vi "Mag_Phase_Calculator (SubVI).vi"(7 "even-angle references":cluster{"r0":dbl, "dr":dbl, "Y":dbl[]}[](array[cluster]) {"r0" format="%.2p"; "dr" format="%.2p"; "Y" format="%.2f"}, 8 "error in (no error)":errorcluster, 9 "view":T2={"dB on? (F)"=FALSE, "unwrap phase? (T)"=TRUE, "unit in degree? (T)"=TRUE}, 10 "speed profile":T1 {"speed [RPM]" format="%.2f"; "time [s]" format="%.2f"}, 11 "Array in":waveform(dbl)[](array[waveform])) -> (0 "error out":errorcluster, 1 "Computed Mag/Phase":cluster{dbl, dbl, dbl, dbl}[](array[cluster]), 2 "RPS (Hz)":dbl, 3 "Data Available":bool)   [LabVIEW 2012]
uses:
  <vilib>/addons/Sound and Vibration/Order Analysis/Tach Process/SubVIs/speed profile.ctl
  <vilib>/addons/Sound and Vibration/Order Analysis/Referece Data Processing/OAT Compensate Even Angle Signal (Even Angle Ref, N Channels).vi
  <vilib>/addons/Sound and Vibration/Order Analysis/Resample Order Tracking/SoundVib_OrderTracking.lvlib
  <vilib>/addons/Sound and Vibration/Order Analysis/Referece Data Processing/SoundVib_RefDataProcess.lvlib
  <vilib>/addons/Sound and Vibration/Order Analysis/Tach Process/SoundVib_TachProcess.lvlib
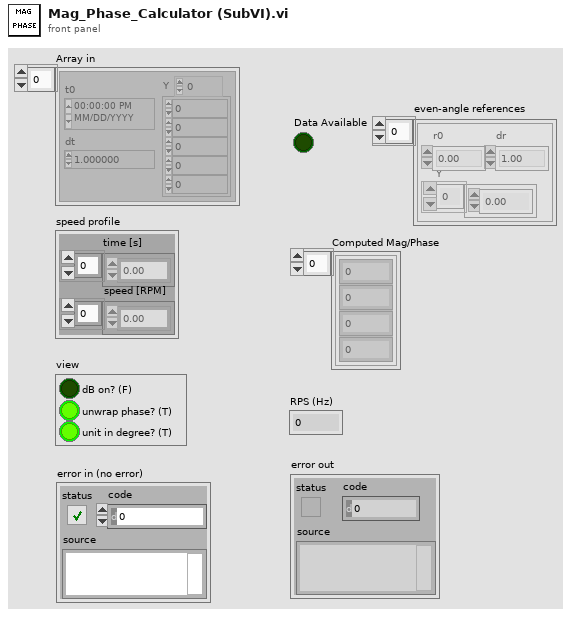
[diagram p1: front panel]
types:
  T1 = typedef "SoundVib_TachProcess.lvlib/speed profile.ctl" = cluster{"time [s]":dbl[], "speed [RPM]":dbl[]}
  T2 = cluster{"dB on? (F)":bool, "unwrap phase? (T)":bool, "unit in degree? (T)":bool}
  T3 = typedef "svc_Resampled Channel Info.ctl" = cluster{"channel name":string, "description":string, " channel info":T4}
  T4 = typedef "svc_Channel Info.ctl" = cluster{"sensor sensitivity [mV/EU]":dbl, "engineering units":T5, "dB reference [EU]":dbl, "custom label":string, "weighting filter":T6, "pregain [dB]":dbl}
  T5 = typedef "svc_Engineering Units Text Ring.ctl" = u16
  T6 = typedef "svc_Weighting Filter Text Ring.ctl" = u16
  T7 = typedef "OAT Position Info.ctl" = cluster{"positions [s]":dbl[], "samples/rev":dbl}
  T8 = cluster{"time/rev/rpm":dbl[], "magnitude":dbl[]}[][]
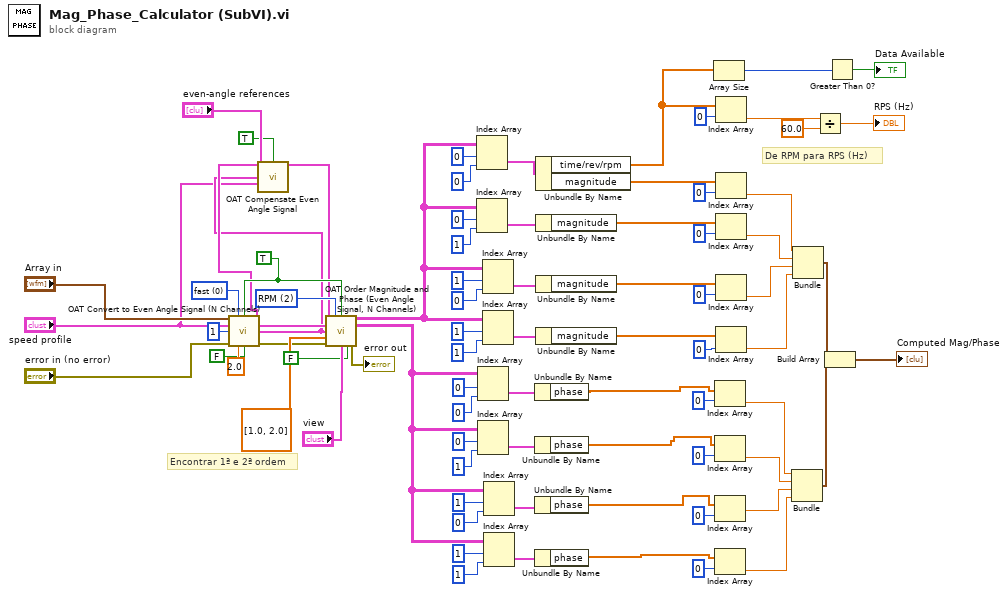
[diagram p0: block diagram]
diagram:
  w79 = TRUE
  w28 = u16 0 items=["fast", "accurate"] ("analysis method")
  w23 = u16 2 items=["Time", "Revolution", "RPM"] ("X axis selection")
  # "Encontrar 1ª e 2ª ordem"
  # "De RPM para RPS (Hz)"
  n1 = call <vilib>:"OAT Convert to Even Angle Signal (N Channels).vi"("scaled signals [EU]"="Array in", "analysis method"=w28, "reset? (F)"=w79, "speed profile"="speed profile", "pulse/revolution (1)"=1, "error in (no error)"="error in (no error)", "max order (auto)"=2.0, "zero delay? (F)"=FALSE) -> ("even-angle signals"=w13:cluster{"r0":dbl, "dr":dbl, "Y":dbl[]}[], "even-angle channel info"=w22:T3[], "even-angle position info"=w11:T7, "error out"=w27:errorcluster)  [unwired: 3 in, 1 out]
  n2 = call-poly <vilib>:"OAT Compensate Even Angle Signal.vi"("even-angle signals"=w13, "reset? (F)"=TRUE, "even-angle references"="even-angle references", "even-angle position info"=w11, "speed profile"="speed profile") -> ("compensated even-angle signals"=w12:cluster{"r0":dbl, "dr":dbl, "Y":dbl[]}[])  [unwired: 7 in, 3 out]
  n3 = call <vilib>:"OAT Order Magnitude and Phase (Even Angle Signal, N Channels).vi"("even-angle signals"=w12, "x-axis selection"=w23, "reset? (F)"=w79, "even-angle channel info"=w22, "even-angle position info"=w11, "orders to compute (1.0)"=dbl[] [1.0, 2.0], "error in (no error)"=w27, "view"="view", "zero delay? (F)"=FALSE) -> ("magnitudes [RMS]"=w3:T8, "phases [phase lag]"=w2:cluster{"time/rev/rpm":dbl[], "phase":dbl[]}[][], "error out"=→"error out":errorcluster)  [unwired: 1 in, 3 out]
  n4 = Index Array(array=w3, index (row)=0, index (col)=0 ("index (row)")) -> (element=w32:cluster{"time/rev/rpm":dbl[], "magnitude":dbl[]})
  n5 = Index Array(array=w3, index (row)=0, index (col)=1 ("index (row)")) -> (element=w35:cluster{"time/rev/rpm":dbl[], "magnitude":dbl[]})
  n6 = Index Array(array=w2, index (row)=0, index (col)=0 ("index (row)")) -> (element=w48:cluster{"time/rev/rpm":dbl[], "phase":dbl[]})
  n7 = Index Array(array=w2, index (row)=0, index (col)=1 ("index (row)")) -> (element=w8:cluster{"time/rev/rpm":dbl[], "phase":dbl[]})
  n8 = Index Array(array=w3, index (row)=1, index (col)=0 ("index (row)")) -> (element=w37:cluster{"time/rev/rpm":dbl[], "magnitude":dbl[]})
  n9 = Index Array(array=w3, index (row)=1, index (col)=1 ("index (row)")) -> (element=w40:cluster{"time/rev/rpm":dbl[], "magnitude":dbl[]})
  n10 = Index Array(array=w2, index (row)=1, index (col)=0 ("index (row)")) -> (element=w44:cluster{"time/rev/rpm":dbl[], "phase":dbl[]})
  n11 = Index Array(array=w2, index (row)=1, index (col)=1 ("index (row)")) -> (element=w41:cluster{"time/rev/rpm":dbl[], "phase":dbl[]})
  n12 = Unbundle By Name(w48) -> ("phase"=w7:dbl[])
  n13 = Unbundle By Name(w8) -> ("phase"=w4:dbl[])
  n14 = Unbundle By Name(w44) -> ("phase"=w6:dbl[])
  n15 = Unbundle By Name(w41) -> ("phase"=w5:dbl[])
  n16 = Unbundle By Name(w32) -> ("time/rev/rpm"=w14:dbl[], "magnitude"=w61:dbl[])
  n17 = Unbundle By Name(w35) -> ("magnitude"=w62:dbl[])
  n18 = Unbundle By Name(w37) -> ("magnitude"=w63:dbl[])
  n19 = Unbundle By Name(w40) -> ("magnitude"=w64:dbl[])
  n20 = Array Size(array=w14) -> (size(s)=w15:i32)
  n21 = Index Array(array=w7, index=0) -> (element=w69:dbl)
  n22 = Index Array(array=w4, index=0) -> (element=w70:dbl)
  n23 = Index Array(array=w6, index=0) -> (element=w71:dbl)
  n24 = Index Array(array=w5, index=0) -> (element=w72:dbl)
  n25 = Index Array(array=w14, index=0) -> (element=w75:dbl)
  n26 = Index Array(array=w61, index=0) -> (element=w65:dbl)
  n27 = Index Array(array=w62, index=0) -> (element=w66:dbl)
  n28 = Index Array(array=w63, index=0) -> (element=w67:dbl)
  n29 = Index Array(array=w64, index=0) -> (element=w68:dbl)
  n30 = Bundle(w69, w70, w71, w72) -> (w74:cluster{dbl, dbl, dbl, dbl})  [unwired: 1 in]
  n31 = Bundle(w65, w66, w67, w68) -> (w73:cluster{dbl, dbl, dbl, dbl})  [unwired: 1 in]
  n32 = Divide(x=w75, y=60.0) -> (x/y=→"RPS (Hz)":dbl)
  n33 = Build Array(w73, w74) -> (→"Computed Mag/Phase":cluster{dbl, dbl, dbl, dbl}[])
  n34 = Greater Than 0?(x=w15) -> (x > 0?=→"Data Available":bool)
